vi "test_lugre_1.vi"() -> ()   [LabVIEW 2012]
panel:
  out "Waveform Chart":dbl(graph)
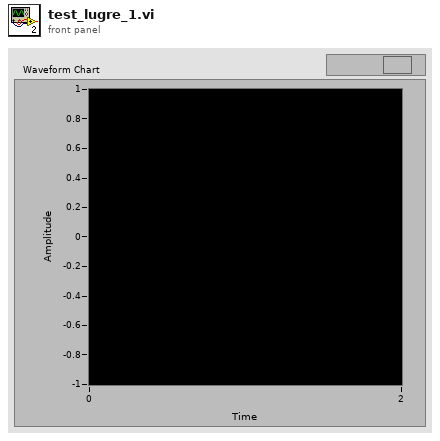
[diagram p1: front panel]
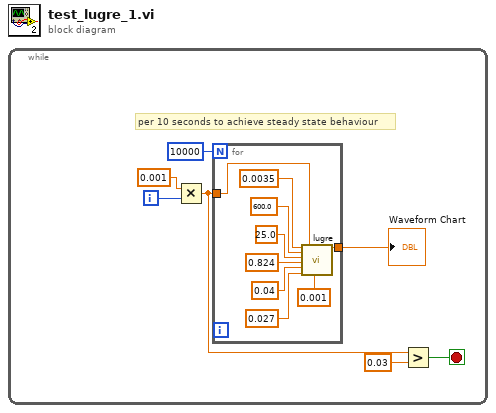
[diagram p0: block diagram]
diagram:
  n1 = while {
    i -> [w6]
    stop <- w3 stop-if-true
    # "per 10 seconds to achieve steady state behaviour"
    n2 = Multiply(x=0.001, y=w6) -> (x*y=w2:dbl)
    n3 = for {
      N: 10000 -> [_]
      tunnel: w2 -> [w10]
      tunnel: [w9] -> w5
      n4 = call "lugre.vi"("stribeck velocity"=0.0035, "bristle stiffness"=600.0, "bristle damping"=25.0, "viscous friction"=0.824, "stiction friction"=0.04, "columb friction"=0.027, "velocity"=w10, "time sampling"=0.001) -> ("F"=w9:dbl)  [unwired: 10 in, 1 out]
    }
    "Waveform Chart" <- w5
    n5 = Greater?(x=w2, y=0.03) -> (0:w3:bool)
  }
